vi "ControllerMain.vi"(8 "Error In":errorcluster, 11 "Control Mode":T4(ring)) -> (0 "Error Out":errorcluster, 3 "Robot Inputs":T3, 4 "Joystick1DevRef":T1={"Device"=enum."USB 1"}, 5 "Stick0 Buttons":bool[](array[boolean]), 6 "Joystick0DevRef":T1={"Device"=enum."USB 1"}, 7 "Stick0 Axes":dbl[](array[numeric]))   [LabVIEW 2017]
uses:
  TeleopCommands.ctl
  <vilib>/Rock Robotics/WPI/Joystick/WPI_JoystickDevRef.ctl
  <vilib>/Rock Robotics/WPI/Joystick/WPI_JoystickDeviceEnum.ctl
  <vilib>/Rock Robotics/WPI/Utilities/WPI_GetSetVariantRefNum.vi
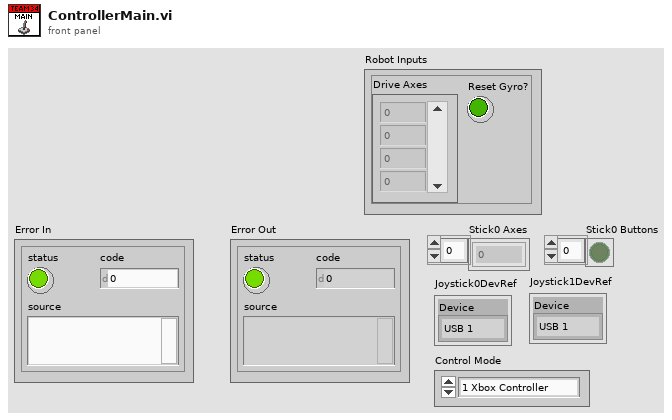
[diagram p1: front panel]
types:
  T1 = typedef "WPI_JoystickDevRef.ctl" = cluster{"Device":T2}
  T2 = typedef "WPI_JoystickDeviceEnum.ctl" = enum16{"USB 0", "USB 1", "USB 2", "USB 3", "USB 4", "USB 5"}
  T3 = typedef "TeleopCommands.ctl" = cluster{"Drive Axes":dbl[], "Reset Gyro?":bool}
  T4 = enum16{"1 Xbox Controller", "2 Xbox Controllers"}
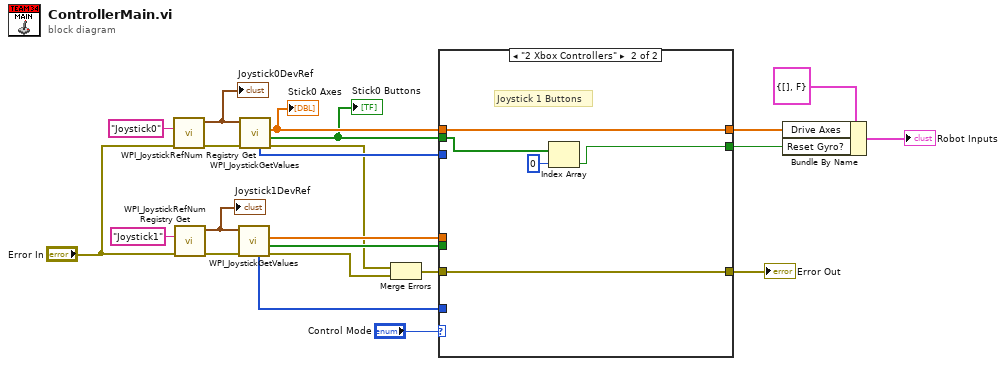
[diagram p0: block diagram]
diagram:
  n1 = call <vilib>:"WPI_JoystickRefNum Registry Get.vi"("error in (no error)"="Error In", "refnum name"="Joystick0") -> ("error out"=w17:errorcluster, "JoystickDevRef"=w22:T1)  [unwired: 8 out]
  "Joystick0DevRef" <- w22
  n2 = call <vilib>:"WPI_JoystickRefNum Registry Get.vi"("error in (no error)"="Error In", "refnum name"="Joystick1") -> ("error out"=w18:errorcluster, "JoystickDevRef"=w19:T1)  [unwired: 8 out]
  "Joystick1DevRef" <- w19
  n3 = call <vilib>:"WPI_JoystickGetValues.vi"("error in (no error)"=w18, "JoystickDevRef"=w19) -> ("error out"=w7:errorcluster, "Buttons"=w13:bool[], "Axes"=w12:dbl[], "POVs"=w4:i16[])  [unwired: 5 in, 1 out]
  n4 = call <vilib>:"WPI_JoystickGetValues.vi"("error in (no error)"=w17, "JoystickDevRef"=w22) -> ("error out"=w8:errorcluster, "Buttons"=w14:bool[], "Axes"=w15:dbl[], "POVs"=w10:i16[])  [unwired: 5 in, 1 out]
  "Stick0 Axes" <- w15
  "Stick0 Buttons" <- w14
  n5 = Merge Errors(w8, w7) -> (w6:errorcluster)
  n6 = case shown="\"2 Xbox Controllers\"" "Control Mode" {
    tunnel: w15 -> [w24 w29]
    tunnel: w14 -> [_ w27]
    tunnel: w13 -> [_ _]
    tunnel: w12 -> [_ _]
    tunnel: [w24 w29] -> w11
    tunnel: w10 -> [_ _]
    tunnel: [w23 w28] -> w5
    tunnel: w6 -> [w23 w28]
    tunnel: w4 -> [_ _]
    tunnel: [_ w25] -> w1
    frame "1 Xbox Controller", Default {
    }
    frame "2 Xbox Controllers" {
      # "Joystick 1 Buttons"
      n7 = Index Array(array=w27, index=0) -> (element=w25:bool)
    }
  }
  "Error Out" <- w5
  n8 = Bundle By Name(cluster=T3 {"Drive Axes"=[], "Reset Gyro?"=FALSE} ("Robot Inputs"), "Drive Axes"=w11, "Reset Gyro?"=w1) -> (→"Robot Inputs":T3)
